vi "Request current CH3 (SubVI).vi"() -> (3 "Request current CH3 / Z":string)   [LabVIEW 2018]
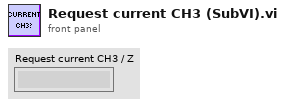
[diagram p1: front panel]
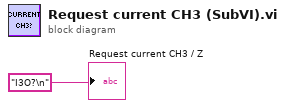
[diagram p0: block diagram]
diagram:
  "Request current CH3 / Z" <- "I3O?\n" ("format string")
